vi "FGV_select inset VI.vi"(4 "Value":variant, 5 "First Run":i32, 6 "Parameter":string, 7 "Function":T1=enum."Get all Opend VIs", 8 "error in (no error)":errorcluster, 9 "Inser VI name":string, 10 "VIs Name":string[](array[string]), 11 "ModulesPath":path) -> (0 "error out":errorcluster, 2 "Inset VI":refnum<vi>)   [LabVIEW 2017]
uses:
  Func_Subpannel.ctl
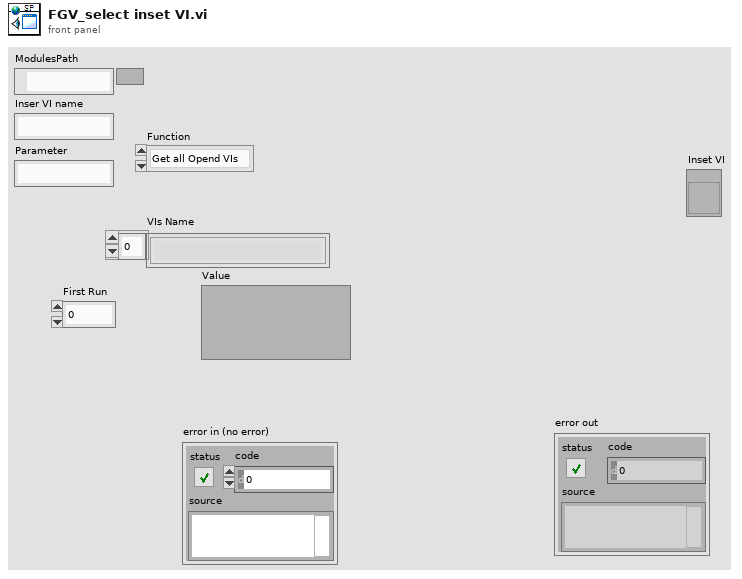
[diagram p1: front panel]
types:
  T1 = typedef "Func_Subpannel.ctl" = enum16{"Initialize", "Get all Opend VIs", "Update Insert VI", "Close all VIs"}
  T2 = cluster{"All VIs":refnum<vi>[], "Insert VI":refnum<vi>}
  T3 = cluster{"Image":path, "Modules":path, "System.ini":path}
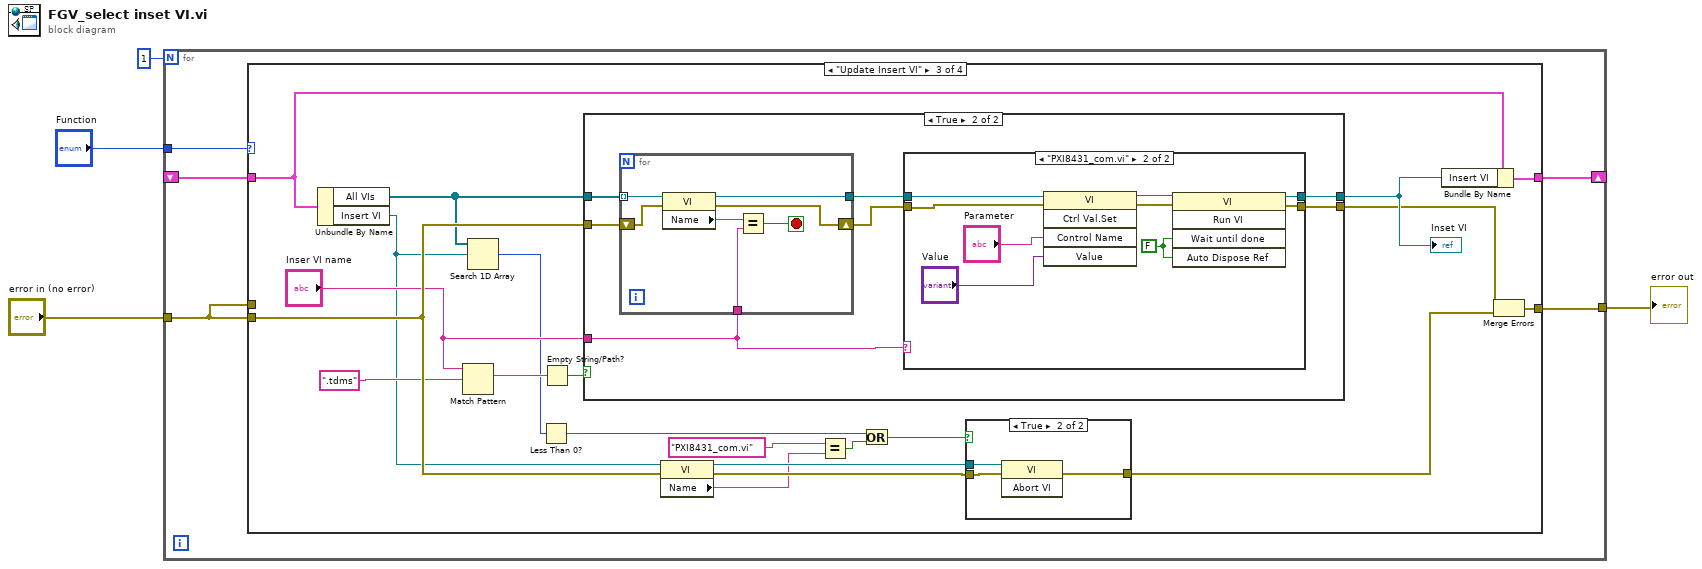
[diagram p0: block diagram]
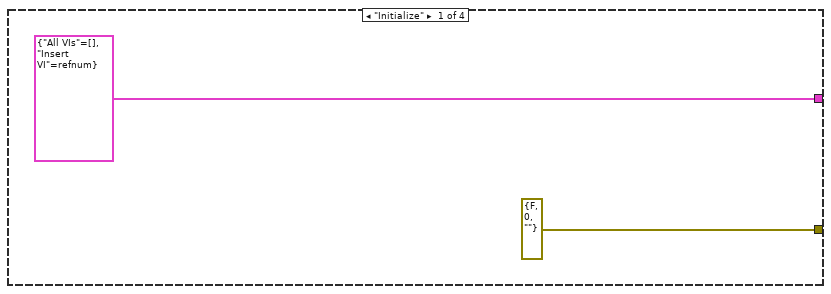
[diagram p2: hidden frame]
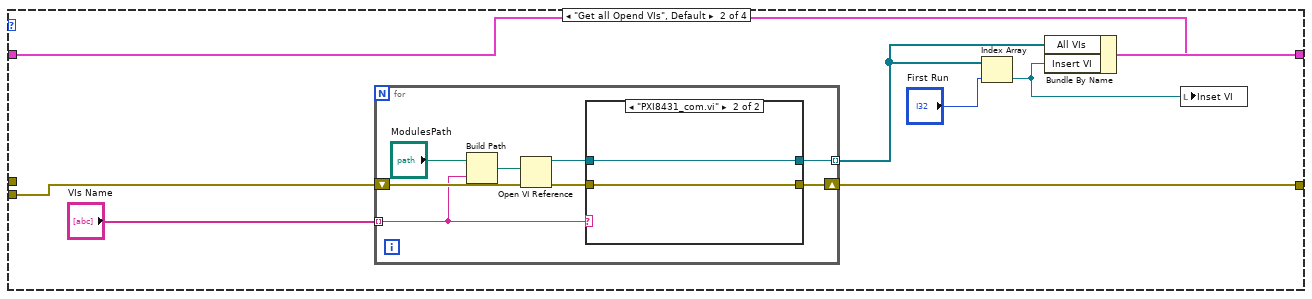
[diagram p3: hidden frame]
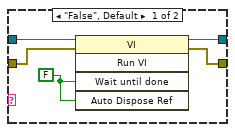
[diagram p4: hidden frame]
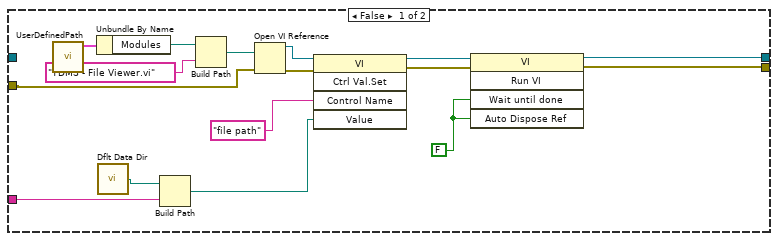
[diagram p5: hidden frame]
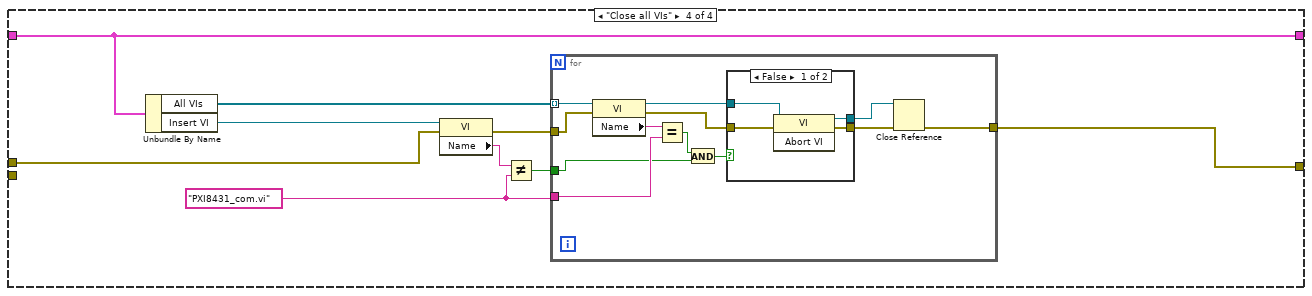
[diagram p8: hidden frame]
diagram:
  n1 = for {
    N: 1 -> [_]
    tunnel: "Function" -> [w9]
    tunnel: [w8] -> w2
    shift-right: [w7] -> _
    shift-left: _ -> [w6]
    tunnel: "error in (no error)" -> [w5]
    n2 = case shown="\"Update Insert VI\"" w9 {
      tunnel: [errorcluster {"status"=FALSE, "code"=0, "source"=""} ("error out") w12 w44 w108] -> w8
      tunnel: [T2 {"All VIs"=[], "Insert VI"=refnum} w16 w54 w109] -> w7
      tunnel: w6 -> [_ w15 w55 w109]
      tunnel: w5 -> [_ w14 w49 _]
      tunnel: w5 -> [_ _ _ w106]
      frame "Initialize" {
      }
      frame "Get all Opend VIs", Default {
        n3 = for {
          tunnel: [w22] -> w17 mode=indexing
          shift-right: [w20] -> w12
          shift-left: w14 -> [w26]
          tunnel: "VIs Name" -> [w24] mode=indexing
          n4 = Build Path(base path="ModulesPath", name or relative path=w24) -> (appended path=w27:path)
          n5 = Open VI Reference(vi path=w27, error in (no error)=w26) -> (vi reference=w23:refnum<vi>, error out=w21:errorcluster)  [unwired: 4 in]
          n6 = case shown="\"PXI8431_com.vi\"" w24 {
            tunnel: w23 -> [w31 w34]
            tunnel: [w30 w34] -> w22
            tunnel: w21 -> [w29 w33]
            tunnel: [w28 w33] -> w20
            frame "False", Default {
              w32 = FALSE
              n7 = invoke class="VI" method="Run VI"(reference=w31, error in=w29, "Wait until done"=w32, "Auto Dispose Ref"=w32) -> (reference out=w30:refnum<vi>, error out=w28:errorcluster)  [unwired: 1 in, 3 out]
            }
            frame "PXI8431_com.vi" {
            }
          }
        }
        n8 = Index Array(array=w17, index="First Run") -> (element=w13:refnum<vi>)
        n9 = Bundle By Name(cluster=w15, "All VIs"=w17, "Insert VI"=w13) -> (w16:T2)
        n10 = local write "Inset VI"(w13) -> ()
      }
      frame "Update Insert VI" {
        n11 = Unbundle By Name(w55) -> ("All VIs"=w42:refnum<vi>[], "Insert VI"=w41:refnum<vi>)
        n12 = Match Pattern(string="Inser VI name", regular expression=".tdms") -> (match substring=w46:string)  [unwired: 1 in, 3 out]
        n13 = Search 1D Array(1D array=w42, element=w41) -> (index of element=w40:i32)  [unwired: 1 in]
        n14 = Less Than 0?(x=w40) -> (x < 0?=w39:bool)
        n15 = Empty String/Path?(string/path=w46) -> (empty?=w47:bool)
        n16 = case shown="True" w47 {
          tunnel: w42 -> [_ w78]
          tunnel: [w56 w76] -> w53
          tunnel: [w57 w75] -> w52
          tunnel: "Inser VI name" -> [w63 w74]
          tunnel: w49 -> [w67 w72]
          frame False {
            w58 = FALSE
            n17 = call "UserDefinedPath.vi"() -> ("ProDefPath"=w71:T3)  [unwired: 11 in]
            n18 = Unbundle By Name(w71) -> ("Modules"=w70:path)
            n19 = call <vilib>:"Dflt Data Dir.vi"() -> ("App:Default Data Directory"=w62:path)
            n20 = Build Path(base path=w62, name or relative path=w63) -> (appended path=w61:path)
            n21 = Build Path(base path=w70, name or relative path="TDMS - File Viewer.vi") -> (appended path=w68:path)
            n22 = Open VI Reference(vi path=w68, error in (no error)=w67) -> (vi reference=w65:refnum<vi>, error out=w66:errorcluster)  [unwired: 4 in]
            n23 = invoke class="VI" method="Ctrl Val.Set"(reference=w65, error in=w66, "Control Name"="file path", "Value"=w61) -> (reference out=w60:refnum<vi>, error out=w59:errorcluster)  [unwired: 1 in, 3 out]
            n24 = invoke class="VI" method="Run VI"(reference=w60, error in=w59, "Wait until done"=w58, "Auto Dispose Ref"=w58) -> (reference out=w56:refnum<vi>, error out=w57:errorcluster)  [unwired: 1 in, 3 out]
          }
          frame True {
            n25 = for {
              shift-right: [w92] -> w73
              shift-left: w72 -> [w95]
              tunnel: w78 -> [w96] mode=indexing
              tunnel: [w91] -> w77
              tunnel: w74 -> [w90]
              stop <- w93 stop-if-true
              n26 = property class="VI"(reference=w96, error in=w95) -> (reference out=w91:refnum<vi>, error out=w92:errorcluster, "Name"=w94:string)
              n27 = Equal?(x=w94, y=w90) -> (x = y?=w93:bool)
            }
            n28 = case shown="\"PXI8431_com.vi\"" w74 {
              tunnel: w77 -> [w80 w89]
              tunnel: w73 -> [w79 w81]
              tunnel: [w80 w85] -> w76
              tunnel: [w79 w84] -> w75
              frame "False", Default {
              }
              frame "PXI8431_com.vi" {
                w88 = FALSE
                n29 = invoke class="VI" method="Ctrl Val.Set"(reference=w89, error in=w81, "Control Name"="Parameter", "Value"="Value") -> (reference out=w87:refnum<vi>, error out=w86:errorcluster)  [unwired: 1 in, 3 out]
                n30 = invoke class="VI" method="Run VI"(reference=w87, error in=w86, "Wait until done"=w88, "Auto Dispose Ref"=w88) -> (reference out=w85:refnum<vi>, error out=w84:errorcluster)  [unwired: 1 in, 3 out]
              }
            }
          }
        }
        "Inset VI" <- w53
        n31 = property class="VI"(reference=w41, error in=w49) -> (reference out=w51:refnum<vi>, error out=w50:errorcluster, "Name"=w37:string)
        n32 = Equal?(x="PXI8431_com.vi", y=w37) -> (x = y?=w38:bool)
        n33 = Or(x=w39, y=w38) -> (x .or. y?=w35:bool)
        n34 = case shown="True" w35 {
          tunnel: w51 -> [_ w100]
          tunnel: [w97 w99] -> w43
          tunnel: w50 -> [w97 w98]
          frame False {
          }
          frame True {
            n35 = invoke class="VI" method="Abort VI"(reference=w100, error in=w98) -> (error out=w99:errorcluster)  [unwired: 1 in, 2 out]
          }
        }
        n36 = Bundle By Name(cluster=w55, "Insert VI"=w53) -> (w54:T2)
        n37 = Merge Errors(w52, w43) -> (w44:errorcluster)
      }
      frame "Close all VIs" {
        w101 = "PXI8431_com.vi"
        n38 = Unbundle By Name(w109) -> ("All VIs"=w105:refnum<vi>[], "Insert VI"=w107:refnum<vi>)
        n39 = property class="VI"(reference=w107, error in=w106) -> (error out=w104:errorcluster, "Name"=w103:string)  [unwired: 1 out]
        n40 = Not Equal?(x=w103, y=w101) -> (x != y?=w102:bool)
        n41 = for {
          tunnel: w105 -> [w118] mode=indexing
          tunnel: [w121] -> w108
          tunnel: w104 -> [w117]
          tunnel: w101 -> [w115]
          tunnel: w102 -> [w110]
          n42 = property class="VI"(reference=w118, error in=w117) -> (reference out=w114:refnum<vi>, error out=w113:errorcluster, "Name"=w116:string)
          n43 = Equal?(x=w116, y=w115) -> (x = y?=w111:bool)
          n44 = And(x=w111, y=w110) -> (x .and. y?=w112:bool)
          n45 = case shown="False" w112 {
            tunnel: [w125 w126] -> w120
            tunnel: [w124 w127] -> w119
            tunnel: w114 -> [w123 w127]
            tunnel: w113 -> [w122 w126]
            frame False {
              n46 = invoke class="VI" method="Abort VI"(reference=w123, error in=w122) -> (reference out=w124:refnum<vi>, error out=w125:errorcluster)  [unwired: 1 in, 1 out]
            }
            frame True {
            }
          }
          n47 = Close Reference(reference=w119, error in (no error)=w120) -> (error out=w121:errorcluster)
        }
      }
    }
  }
  "error out" <- w2
